vi "Copy Template Library.vi"(0 "Configuration":T1, 11 "error in (no error)":errorcluster) -> (4 "project ref out":refnum<vi>, 15 "error out":errorcluster)   [LabVIEW 2021, in "G-Plugin Editor.lvlib"]
uses:
  G-Plugin Editor.lvlib
  controls/Data Holder.ctl
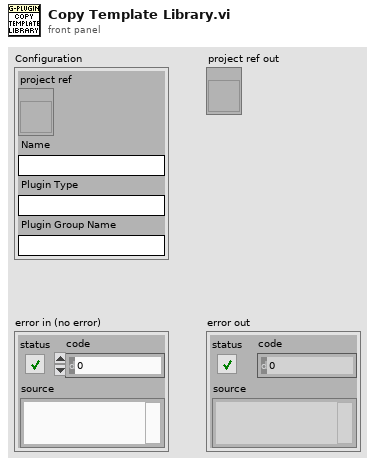
[diagram p1: front panel]
types:
  T1 = typedef "G-Plugin Editor.lvlib/Data Holder.ctl" = cluster{"project ref":refnum<vi>, "Name":string, "Plugin Type":string, "Plugin Group Name":string}
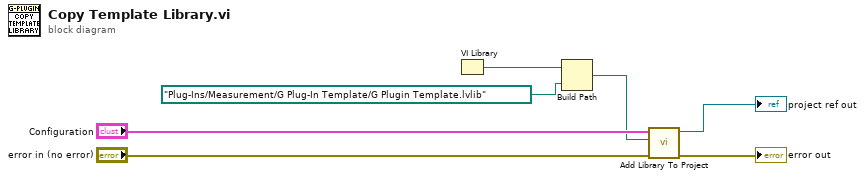
[diagram p0: block diagram]
diagram:
  n1 = VI Library() -> (path=w3:path)
  n2 = Build Path(base path=w3, name or relative path=path "Plug-Ins/Measurement/G Plug-In Template/G Plugin Template.lvlib") -> (appended path=w1:path)
  n3 = call "Add Library To Project.vi"("error in"="error in (no error)", "library path"=w1, "Config"="Configuration") -> ("error out"=→"error out":errorcluster, "project ref out"=→"project ref out":refnum<vi>)  [unwired: 7 in]
